vi "Agilent 2000 3000 X-Series Acquire Waveform.vi"(9 "Maximum Time (10000 ms)":u32=10000, 10 "Auto Scale Source (0: Channel 1)":i32(ring) items=["Channel 1"=0, "Channel 2"=1, "Channel 3"=2, "Channel 4"=3, "Digital Bus Low"=9, "Digital Bus High"=10], 11 "VISA resource name":refnum<visa-resource-name>) -> (3 "Waveform Data":waveform(dbl)(graph))   [LabVIEW 2018]
doc: "This example shows how to use autosetup and acquire a waveform on a single channel."
uses:
  <instrlib>/Agilent 2000 3000 X-Series/Agilent 2000 3000 X-Series.lvlib
panel:
  # "(c) 2011-2018 National Instruments.  ALL RIGHTS RESERVED."
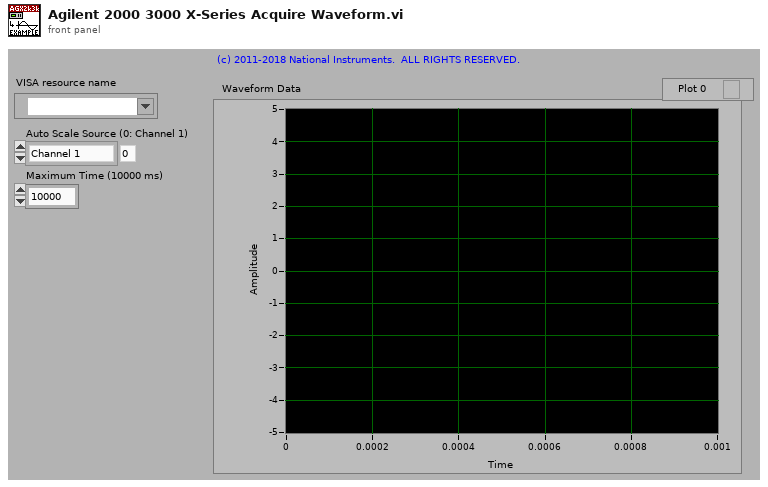
[diagram p1: front panel]
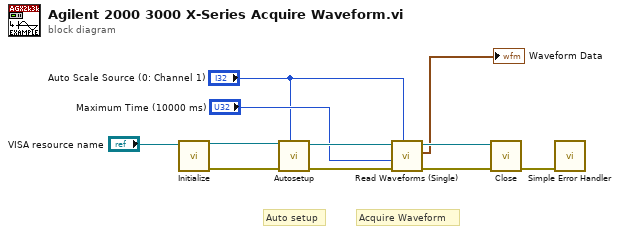
[diagram p0: block diagram]
diagram:
  # "Acquire Waveform"
  # "Auto setup"
  n1 = call <instrlib>:"Initialize.vi"("VISA resource name"="VISA resource name") -> ("error out"=w9:errorcluster, "VISA resource name out"=w8:refnum<visa-resource-name>)  [unwired: 4 in, 5 out]
  n2 = call <instrlib>:"Autosetup.vi"("Auto Scale Source (0: Channel 1)"="Auto Scale Source (0: Channel 1)", "error in (no error)"=w9, "VISA resource name"=w8) -> ("error out"=w4:errorcluster, "VISA resource name out"=w5:refnum<visa-resource-name>)  [unwired: 3 in, 4 out]
  n3 = call <instrlib>:"Read Waveforms (Single).vi"("Bind Source Channel (2: None)"="Auto Scale Source (0: Channel 1)", "error in (no error)"=w4, "Timeout (10000 ms)"="Maximum Time (10000 ms)", "VISA resource name"=w5) -> ("error out"=w7:errorcluster, "Waveform Data"=→"Waveform Data":waveform(dbl), "VISA resource name out"=w6:refnum<visa-resource-name>)  [unwired: 1 in, 4 out]
  n4 = call <instrlib>:"Close.vi"("error in (no error)"=w7, "VISA resource name"=w6) -> ("error out"=w11:errorcluster)  [unwired: 9 out]
  n5 = call <vilib>:"Simple Error Handler.vi"("error in (no error)"=w11) -> ()  [unwired: 1 in, 8 out]
